vi "Pane Relief UI.vi"(8 "Error In":errorcluster, 11 "QD Launch VI Ref":refnum<vi>) -> (0 "Error Out":errorcluster)   [LabVIEW 2017]
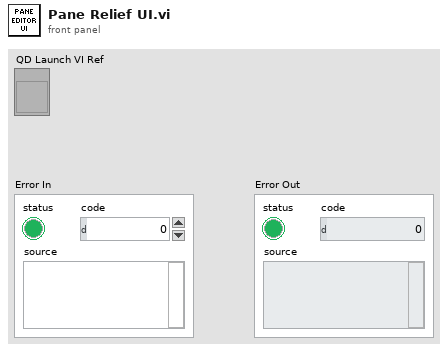
[diagram p1: front panel]
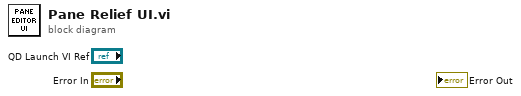
[diagram p0: block diagram]
diagram:
